vi "Slug Test.vi"(9 "# SS":i32=10, 11 "Output File":path) -> ()   [LabVIEW 2016]
uses:
  ad interface/Global_SIM_switch.vi
  <vilib>/Utility/file.llb/Write To Spreadsheet File (DBL).vi
panel:
  out "Timestamp(ms)":u32
  in  "exit":bool
  out "logging_active":bool
  in  "Log control":bool
  in  "Loop period (ms)":u32=1000
  out "Start_log_Timestamp(ms)":u32=8371000
  out "Corrected Pressure":dbl(graph)=0.0045502279410536885
  out "Pressure":dbl(graph)=-28.805587314601613
  out "IK":dbl(graph)=14.983645719671062
  out "Flow":dbl(graph)=19.134611187173405
  out "K":i32(graph)=10
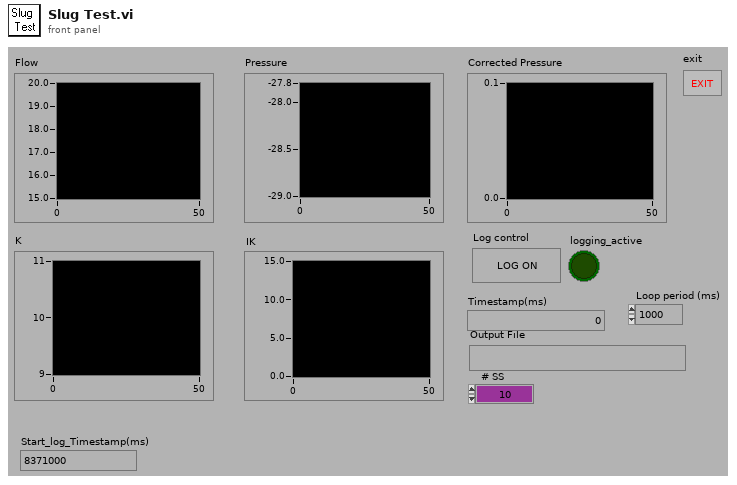
[diagram p1: front panel]
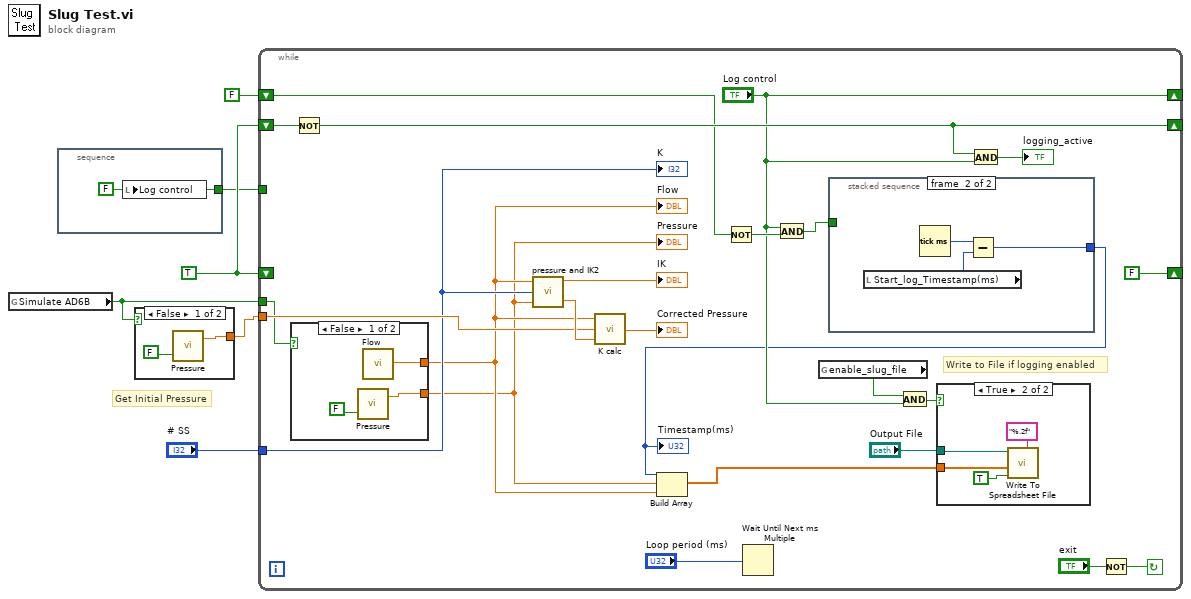
[diagram p0: block diagram]
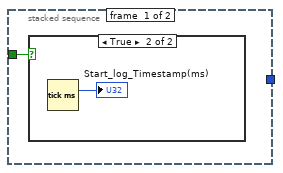
[diagram p2: hidden frame]
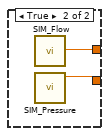
[diagram p5: hidden frame]
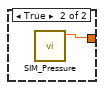
[diagram p6: hidden frame]
diagram:
  w3 = TRUE
  # "Get Initial Pressure"
  n1 = global read "Global_SIM_switch.vi" "Simulate AD6B"() -> (w4:bool)
  n2 = stacked-sequence {
    tunnel: [w7] -> w1
    frame #0 {
      w7 = FALSE ("Log control")
      n3 = local write "Log control"(w7) -> ()
    }
  }
  n4 = case shown="False" w4 {
    tunnel: [w9 w10] -> w5
    frame False {
      n5 = call "Pressure.vi"("Zero Pressure\n(F = leave as is)"=FALSE ("Zero Pressure\n(F = leave as is)")) -> ("Pressure"=w9:dbl)  [unwired: 2 in]
    }
    frame True {
      n6 = call "SIM_Pressure.vi"() -> ("Pressure"=w10:dbl)  [unwired: 11 in]
    }
  }
  n7 = while {
    shift-right: [FALSE] -> _
    shift-left: w3 -> [_]
    tunnel: "# SS" -> [w28]
    tunnel: w5 -> [w31]
    tunnel: w4 -> [w30]
    shift-right: [w23] -> _
    shift-left: w3 -> [w25]
    shift-right: ["Log control"] -> _
    shift-left: FALSE ("Log control") -> [w15]
    tunnel: w1 -> [_]
    stop <- w21 continue-if-true
    # "Write to File if logging enabled"
    n8 = case shown="False" w30 {
      tunnel: [w46 w48] -> w27
      tunnel: [w45 w47] -> w26
      frame False {
        n9 = call "Pressure.vi"("Zero Pressure\n(F = leave as is)"=FALSE ("Zero Pressure\n(F = leave as is)")) -> ("Pressure"=w45:dbl)  [unwired: 2 in]
        n10 = call "Flow.vi"() -> ("Flow (ml/min)"=w46:dbl)  [unwired: 3 in]
      }
      frame True {
        n11 = call "SIM_Flow.vi"() -> ("Flow (ml/min)"=w48:dbl)  [unwired: 3 in]
        n12 = call "SIM_Pressure.vi"() -> ("Pressure"=w47:dbl)  [unwired: 11 in]
      }
    }
    "Pressure" <- w26
    "Flow" <- w27
    n13 = Not(x=w25) -> (.not. x?=w23:bool)
    n14 = call "pressure and IK2.vi"("Pressure"=w26, "Ft. of SS"=w28, "flow"=w27) -> ("Corrected Headloss"=w32:dbl, "IK"=→"IK":dbl)
    n15 = call "K calc.vi"("Current Head"=w32, "Initial Head"=w31, "Flow"=w27) -> ("K"=→"Corrected Pressure":dbl)
    n16 = Not(x=w15) -> (.not. x?=w14:bool)
    n17 = Wait Until Next ms Multiple(millisecond multiple="Loop period (ms)") -> ()  [unwired: 1 out]
    n18 = And(x="Log control", y=w14) -> (x .and. y?=w13:bool)
    n19 = global read "Global_SIM_switch.vi" "enable_slug_file"() -> (w17:bool)
    n20 = stacked-sequence {
      tunnel: w13 -> [w35 _]
      tunnel: [_ w37] -> w11
      frame #0 {
        n21 = case shown="True" w35 {
          frame False {
          }
          frame True {
            n22 = Tick Count (ms)() -> (millisecond timer value=→"Start_log_Timestamp(ms)":u32)
          }
        }
      }
      frame #1 {
        n23 = local read "Start_log_Timestamp(ms)"() -> (w38:u32)
        n24 = Tick Count (ms)() -> (millisecond timer value=w39:u32)
        n25 = Subtract(x=w39, y=w38) -> (x-y=w37:u32)
      }
    }
    "Timestamp(ms)" <- w11
    n26 = Build Array(w11, w26, w27) -> (w20:dbl[])
    n27 = And(x=w17, y="Log control") -> (x .and. y?=w18:bool)
    n28 = case shown="True" w18 {
      tunnel: w20 -> [_ w40]
      tunnel: "Output File" -> [_ w43]
      frame False {
      }
      frame True {
        n29 = call-poly <vilib>:"Write To Spreadsheet File.vi"("format (%.3f)"="%.2f", "append to file? (new file:F)"=TRUE, "1D data"=w40, "file path (dialog if empty)"=w43) -> ()  [unwired: 4 in, 1 out]
      }
    }
    n30 = And(x=w23, y="Log control") -> (x .and. y?=→"logging_active":bool)
    n31 = Not(x="exit") -> (.not. x?=w21:bool)
    "K" <- w28
  }
